vi "deleteTuplaEnDBVarilla.vi"(8 "error in":errorcluster, 11 "claseVarilla in":refnum<class "claseVarilla.lvclass">) -> (0 "error out":errorcluster, 3 "claseVarilla out":refnum<class "claseVarilla.lvclass">)   [LabVIEW 2014, in "claseVarilla.lvclass"]
uses:
  claseVarilla.lvclass
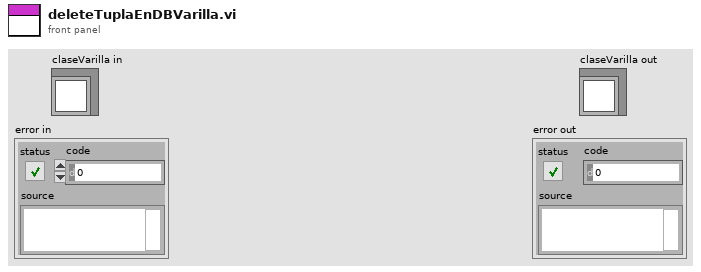
[diagram p1: front panel]
types:
  T1 = cluster{"idRod":dbl, "camposDeMedicion":string, "dateCreate":timestamp, "idProduct":dbl, "idImage":dbl}
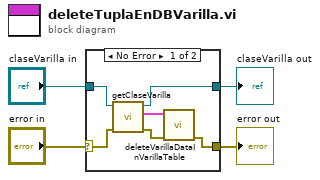
[diagram p0: block diagram]
diagram:
  n1 = case shown="No Error" "error in" {
    selector: "error in" -> [w8 w12]
    tunnel: [w7 w12] -> w3
    tunnel: [w5 w11] -> w2
    tunnel: "claseVarilla in" -> [w6 w11]
    frame No Error {
      n2 = call "getClaseVarilla.vi"("error in"=w8, "claseVarilla in"=w6) -> ("error out"=w9:errorcluster, "dataReading"=w10:T1, "claseVarilla out"=w5:refnum<class "claseVarilla.lvclass">)  [unwired: 7 in]
      n3 = call "deleteVarillaDataInVarillaTable.vi"("error in"=w9, "dataReadingToDelete"=w10) -> ("error out"=w7:errorcluster)  [unwired: 9 in]
    }
    frame Error {
    }
  }
  "claseVarilla out" <- w2
  "error out" <- w3
